vi "S2C_ExeScriptResult.vi"(8 "Error In":errorcluster, 10 "Measurement":string, 11 "Q_Ref":refnum<queue>) -> (0 "Error Out":errorcluster)   [LabVIEW 2015]
doc: "Updates the execution table for auto-scrolling, determines the current line item result, and determines the next step to take in the execution."
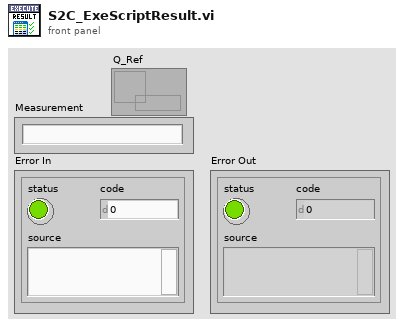
[diagram p1: front panel]
types:
  T1 = typedef "S2C_ResultStatus.ctl" = enum16{"Passed", "Failed", "Logged", "Aborted", "Error", "Testing...", "Paused", "No Record"}
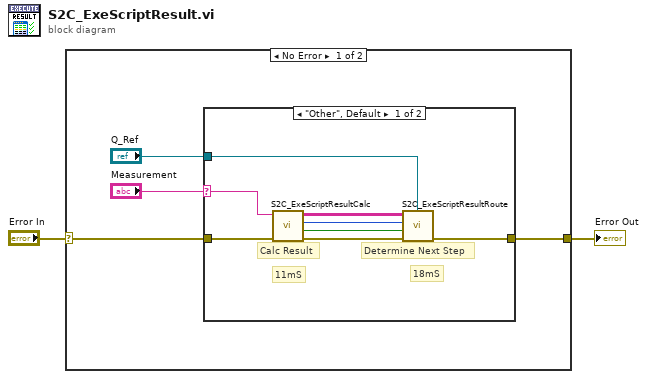
[diagram p0: block diagram]
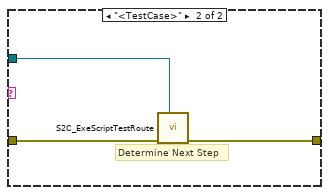
[diagram p2: hidden frame]
diagram:
  n1 = case shown="No Error" "Error In" {
    selector: "Error In" -> [w6 w18]
    tunnel: [w5 w18] -> w1
    frame No Error {
      n2 = case shown="\"Other\", Default" "Measurement" {
        selector: "Measurement" -> [w11 _]
        tunnel: w6 -> [w9 w17]
        tunnel: [w7 w16] -> w5
        tunnel: "Q_Ref" -> [w14 w15]
        frame "Other", Default {
          # "18mS"
          # "11mS"
          # "Determine Next Step"
          # "Calc Result"
          n3 = call "S2C_ExeScriptResultCalc.vi"("Error In"=w9, "Measurement"=w11) -> ("Error Out"=w8:errorcluster, "LastMeas?"=w12:bool, "Result"=w13:T1, "Data"=w10:string[][])  [unwired: 6 in]
          n4 = call "S2C_ExeScriptResultRoute.vi"("Q_Ref"=w14, "Error In"=w8, "LastMeas?"=w12, "Result"=w13, "Data In"=w10) -> ("Error Out"=w7:errorcluster)  [unwired: 6 in]
        }
        frame "<TestCase>" {
          # "Determine Next Step"
          n5 = call "S2C_ExeScriptTestRoute.vi"("Q_Ref"=w15, "Error In"=w17) -> ("Error Out"=w16:errorcluster)  [unwired: 9 in]
        }
      }
    }
    frame Error {
    }
  }
  "Error Out" <- w1
